vi "PASCO_PID.vi"(0 "Desired Rate":dbl(slide) scale=0.0..1.0, 5 "Actual Rate":dbl, 7 "Loop Iterations":i32, 9 "Integral Reset":bool, 12 "P Gain":dbl=1.0, 13 "I Gain":dbl=0.01, 14 "D Gain":dbl) -> (4 "Output":dbl, 15 "Array Data":dbl[](graph))   [LabVIEW 2011]
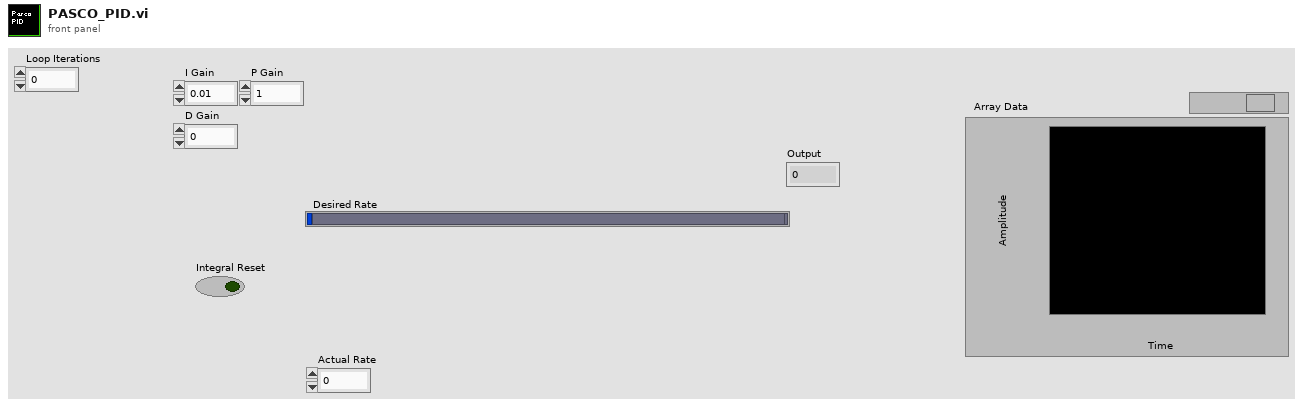
[diagram p1: front panel]
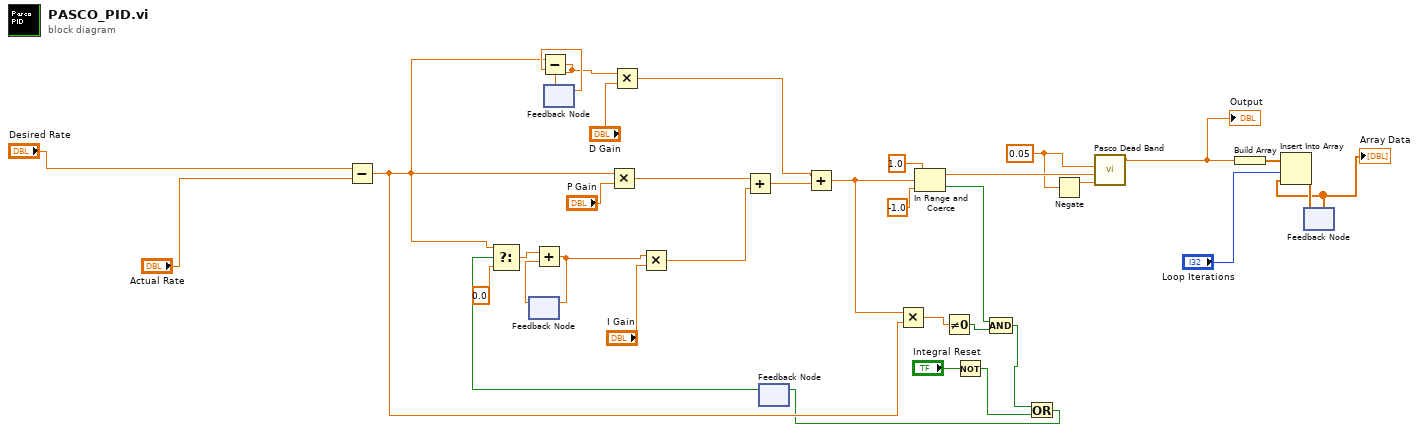
[diagram p0: block diagram]
diagram:
  w14 = 0.05 ("upper limit")
  n1 = Subtract(x="Desired Rate", y="Actual Rate") -> (x-y=w17:dbl)
  n2 = feedback #1() -> (w30:dbl)  [unwired: 1 in]
  n3 = feedback #2() -> (w29:dbl)  [unwired: 1 in]
  n4 = Subtract(x=w17, y=w29) -> (x-y=w28:dbl)
  n5 = feedback-in #2(w28) -> ()
  n6 = Multiply(x=w17, y="P Gain") -> (x*y=w9:dbl)
  n7 = Multiply(x=w28, y="D Gain") -> (x*y=w20:dbl)
  n8 = feedback #3() -> (w12:bool)  [unwired: 1 in]
  n9 = Select(t=w17, s=w12, f=0.0) -> (s? t:f=w22:dbl)
  n10 = Add(x=w22, y=w30) -> (x+y=w10:dbl)
  n11 = feedback-in #1(w10) -> ()
  n12 = Multiply(x=w10, y="I Gain") -> (x*y=w8:dbl)
  n13 = Add(x=w9, y=w8) -> (x+y=w19:dbl)
  n14 = Add(x=w20, y=w19) -> (x+y=w18:dbl)
  n15 = Multiply(x=w18, y=w17) -> (x*y=w26:dbl)
  n16 = In Range and Coerce(upper limit=1.0, x=w18, lower limit=-1.0) -> (coerced(x)=w16:dbl, In Range?=w24:bool)
  n17 = Not Equal To 0?(x=w26) -> (x != 0?=w25:bool)
  n18 = Not(x="Integral Reset") -> (.not. x?=w2:bool)
  n19 = Compound Arithmetic op=AND(w24, w25) -> (w3:bool)
  n20 = Or(x=w3, y=w2) -> (x .or. y?=w1:bool)
  n21 = feedback-in #3(w1) -> ()
  n22 = Negate(x=w14) -> (-x=w15:dbl)
  n23 = call "Pasco Dead Band.vi"("lower limit"=w15, "PWM Power"=w16, "upper limit"=w14) -> ("PWM Power"=w13:dbl)  [unwired: 7 in, 1 out]
  "Output" <- w13
  n24 = Build Array(w13) -> (w33:dbl[])
  n25 = feedback #4() -> (w21:dbl[])  [unwired: 1 in]
  "Array Data" <- w21
  n26 = Insert Into Array(array=w33, index="Loop Iterations", new element=w21) -> (w32:dbl[])
  n27 = feedback-in #4(w32) -> ()
